vi "Verify Multi Combos.vi"(8 "error in":errorcluster) -> (0 "error out":errorcluster)   [LabVIEW 2020, in "Caraya Extension Tests.lvclass"]
uses:
  Caraya Extension Tests.lvclass
  e89fde1e-082c-4af0-b21f-ce2027384817.vi
  1ea2ceb1-3819-4dd0-8a62-7a1566423357.vi
  f0b51538-8a42-4750-ab89-e9f14ef91f99.vi
  Source/Extensions/Caraya.Extension/Caraya.Extension.lvlib
  <vilib>/addons/_JKI Toolkits/Caraya/classes/Test/Test.lvclass
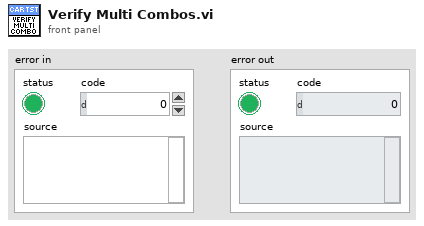
[diagram p1: front panel]
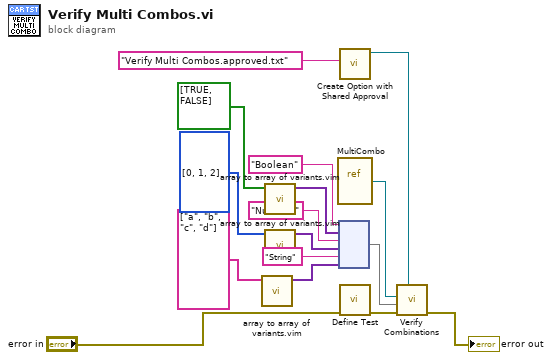
[diagram p0: block diagram]
diagram:
  n1 = call "array to array of variants.vim"("Array in"=string[] ["a", "b", "c", "d"]) -> ("Array out"=w5:variant[])  [unwired: 10 in]
  n2 = call "array to array of variants.vim"("Array in"=bool[] [TRUE, FALSE]) -> ("Array out"=w10:variant[])  [unwired: 10 in]
  n3 = call "array to array of variants.vim"("Array in"=i32[] [0, 1, 2]) -> ("Array out"=w6:variant[])  [unwired: 10 in]
  n4 = vi-ref "MultiCombo.vi"() -> (w8:refnum<vi>)
  n5 = node ("Build Map")("Boolean" ("key"), w10, "Numeric" ("key"), w6, "String" ("key"), w5) -> (w9:map{string, variant[]})
  n6 = call "Create Option with Shared Approval.vi"("Filename"="Verify Multi Combos.approved.txt") -> ("Options outs"=w1:refnum<class "Options.lvclass">)  [unwired: 10 in]
  n7 = call <vilib>:"Define Test.vi"("error in (no error)"="error in") -> ("error out"=w16:errorcluster)  [unwired: 9 in, 1 out]
  n8 = call "Verify Combinations.vi"("Options"=w1, "error in"=w16, "ctl label -> value var[]"=w9, "VI Refnum"=w8) -> ("error out"=→"error out":errorcluster)  [unwired: 6 in, 1 out]
